vi "Evaluate Test Results.vi"(8 "error in (no error)":errorcluster, 9 "Serial Number":string, 10 "Test Configuration":T1, 11 "Test Results":T8) -> (0 "error out":errorcluster, 1 "Summary Out":string[][](array[string]), 2 "Vacuum Results":string[][](array[string]), 3 "Helium Results":string[][](array[string]), 5 "Report Name":string)   [LabVIEW 2014]
uses:
  Tests/Controls/Test Results.ctl
  Tests/Controls/Step Result.ctl
  Tests/Controls/Test Configuration.ctl
  Tests/Controls/Vacuum Test.ctl
  Tests/Controls/Test Timing.ctl
  Tests/Controls/Vaccum Thresholds.ctl
  Tests/Controls/Helium Test.ctl
  Tests/Controls/Helium Thresholds.ctl
  Tests/Controls/Functional Test.ctl
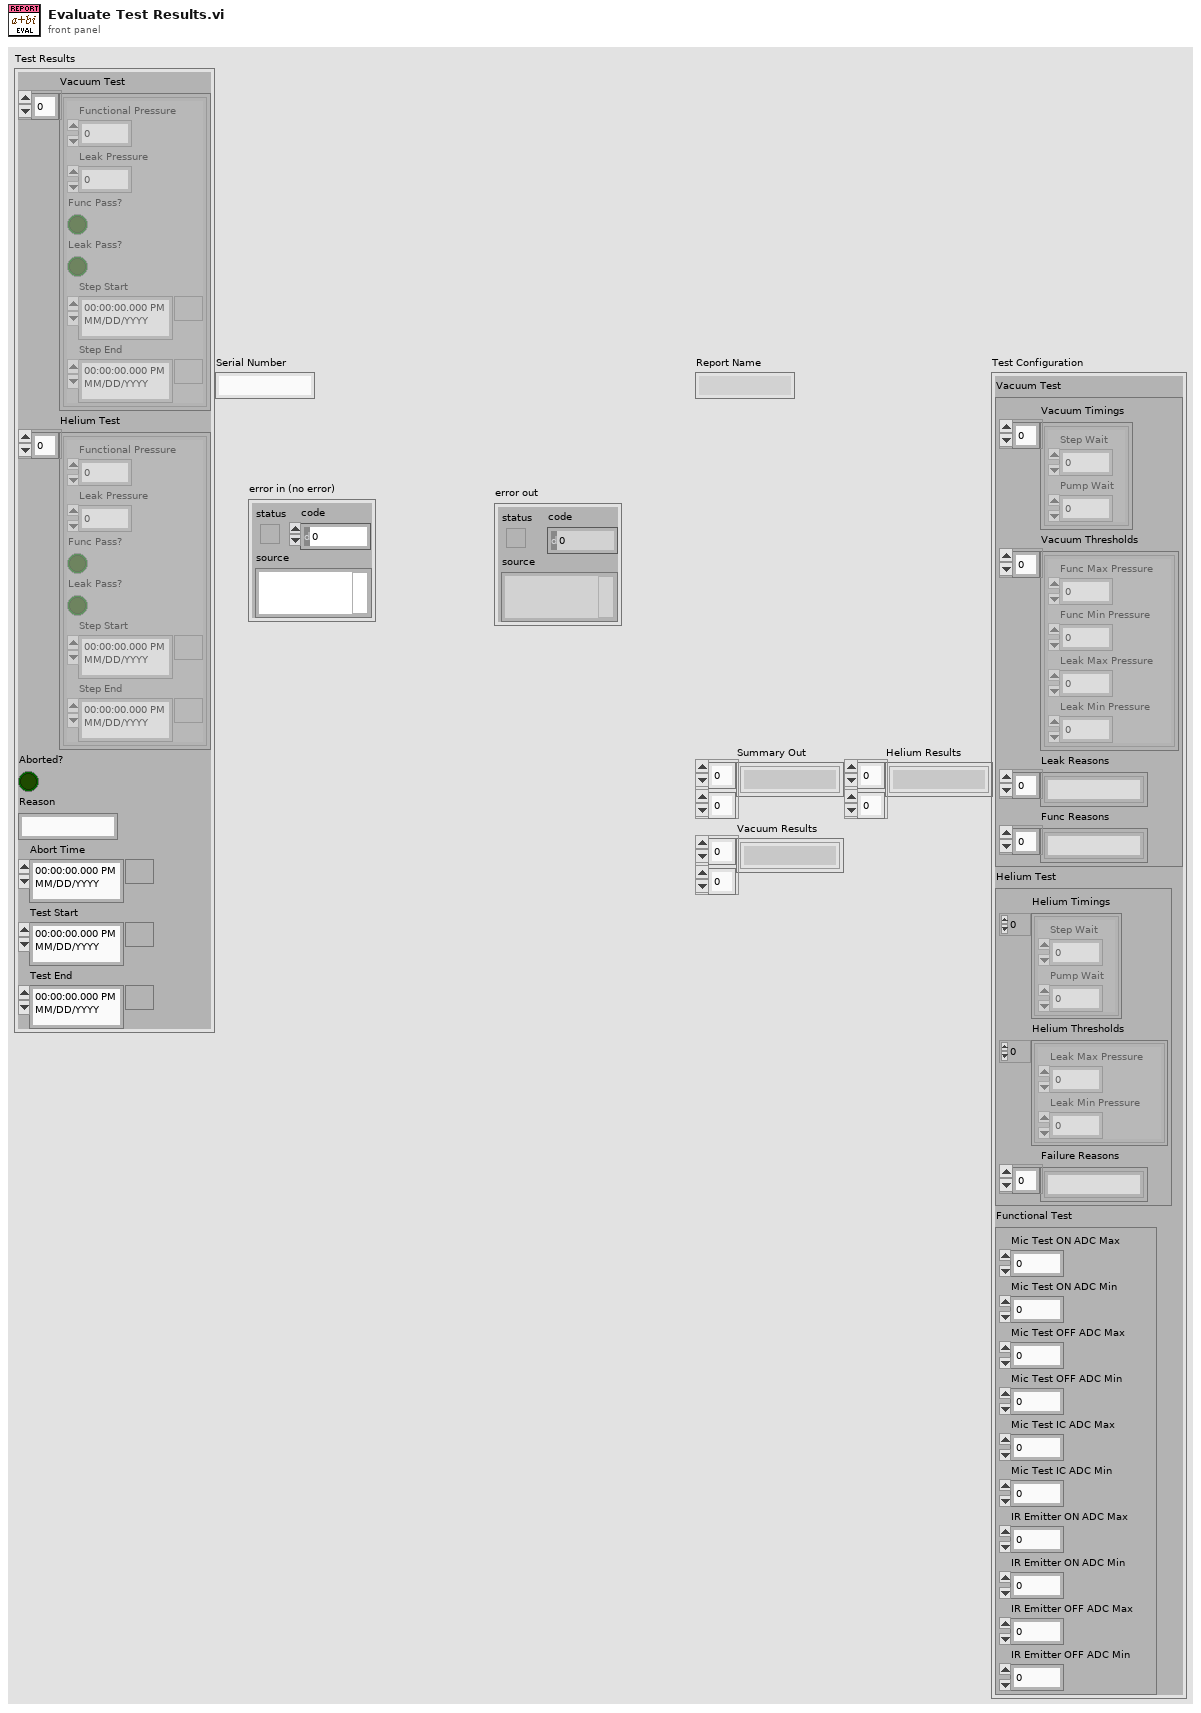
[diagram p1: front panel]
types:
  T1 = typedef "Test Configuration.ctl" = cluster{"Vacuum Test":T2, "Helium Test":T5, "Functional Test":T7}
  T2 = typedef "Vacuum Test.ctl" = cluster{"Vacuum Timings":T3[], "Vacuum Thresholds":T4[], "Leak Reasons":string[], "Func Reasons":string[]}
  T3 = typedef "Test Timing.ctl" = cluster{"Step Wait":dbl, "Pump Wait":dbl}
  T4 = typedef "Vaccum Thresholds.ctl" = cluster{"Func Max Pressure":dbl, "Func Min Pressure":dbl, "Leak Max Pressure":dbl, "Leak Min Pressure":dbl}
  T5 = typedef "Helium Test.ctl" = cluster{"Helium Timings":T3[], "Helium Thresholds":T6[], "Failure Reasons":string[]}
  T6 = typedef "Helium Thresholds.ctl" = cluster{"Leak Max Pressure":dbl, "Leak Min Pressure":dbl}
  T7 = typedef "Functional Test.ctl" = cluster{"Mic Test ON ADC Max":dbl, "Mic Test ON ADC Min":dbl, "Mic Test OFF ADC Max":dbl, "Mic Test OFF ADC Min":dbl, "Mic Test IC ADC Max":dbl, "Mic Test IC ADC Min":dbl, "IR Emitter ON ADC Max":dbl, "IR Emitter ON ADC Min":dbl, "IR Emitter OFF ADC Max":dbl, "IR Emitter OFF ADC Min":dbl}
  T8 = typedef "Test Results.ctl" = cluster{"Vacuum Test":T9[], "Helium Test":T9[], "Aborted?":bool, "Reason":string, "Abort Time":timestamp, "Test Start":timestamp, "Test End":timestamp}
  T9 = typedef "Step Result.ctl" = cluster{"Functional Pressure":dbl, "Leak Pressure":dbl, "Func Pass?":bool, "Leak Pass?":bool, "Step Start":timestamp, "Step End":timestamp}
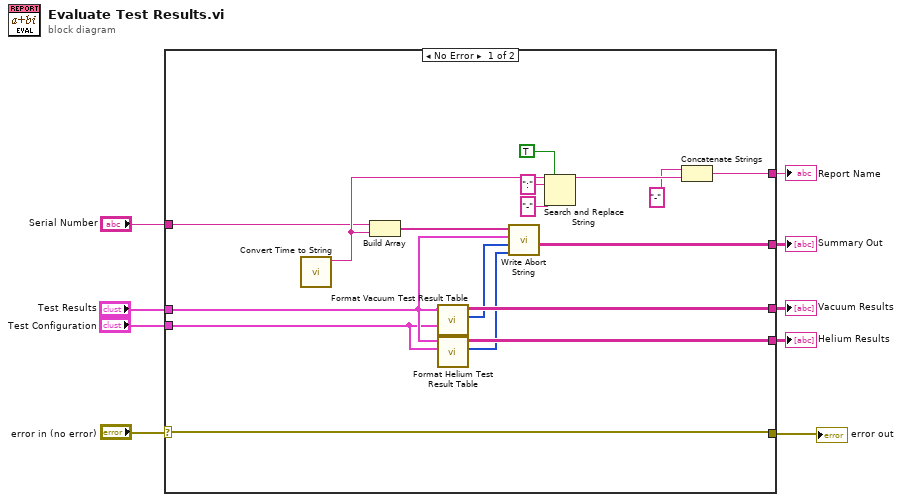
[diagram p0: block diagram]
diagram:
  n1 = case shown="No Error" "error in (no error)" {
    selector: "error in (no error)" -> [w25 w27]
    tunnel: [w25 w27] -> w9
    tunnel: "Test Results" -> [w20 _]
    tunnel: "Test Configuration" -> [w10 _]
    tunnel: [w24 _] -> w5
    tunnel: [w23 _] -> w4
    tunnel: [w19 _] -> w6
    tunnel: [w13 _] -> w3
    tunnel: "Serial Number" -> [w11 _]
    frame No Error {
      n2 = call "Convert Time to String.vi"() -> ("date/time string"=w18:string)  [unwired: 11 in]
      n3 = Build Array(w11, w18) -> (w26:string[])
      n4 = call "Format Vacuum Test Result Table.vi"("Test Configuration"=w10, "Test Results"=w20) -> ("Failure Indexes"=w22:i32[], "Vacuum Results"=w24:string[][])  [unwired: 8 in]
      n5 = call "Format Helium Test Result Table.vi"("Test Configuration"=w10, "Test Results"=w20) -> ("Failure Indexes"=w21:i32[], "Helium Results"=w23:string[][])  [unwired: 8 in]
      n6 = call "Write Abort String.vi"("Helium Fail"=w21, "Vacuum Fail"=w22, "Test Results"=w20, "Summary In"=w26) -> ("Summary Out"=w19:string[][])  [unwired: 7 in]
      n7 = Search and Replace String(replace all?=TRUE ("replace all? (F)"), input string=w18, search string=":", replace string="-" ("replace string (\"\")")) -> (result string=w14:string)  [unwired: 4 in, 3 out]
      n8 = Concatenate Strings("-" ("string"), w14) -> (w13:string)
    }
    frame Error {
    }
  }
  "error out" <- w9
  "Summary Out" <- w6
  "Vacuum Results" <- w5
  "Helium Results" <- w4
  "Report Name" <- w3
